vi "TCP-IP-RaspberryPi.vi"() -> ()   [LabVIEW 2021]
panel:
  out "min value":dbl
  out "max value":dbl
  in  "clear":bool
  in  "save":bool
  out "all values":dbl[](array[numeric])
  out "average":dbl format="%#_5g"
  in  "warning":dbl
  in  "danger":dbl
  out "NORMAL":bool
  out "DANGER":bool
  out "WARNING":bool
  out "Temperature":dbl(graph)
  in  "stop":bool
  out "temperature":dbl
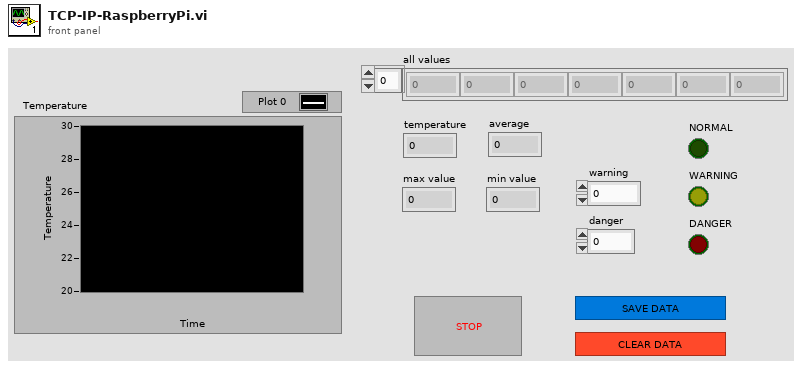
[diagram p1: front panel]
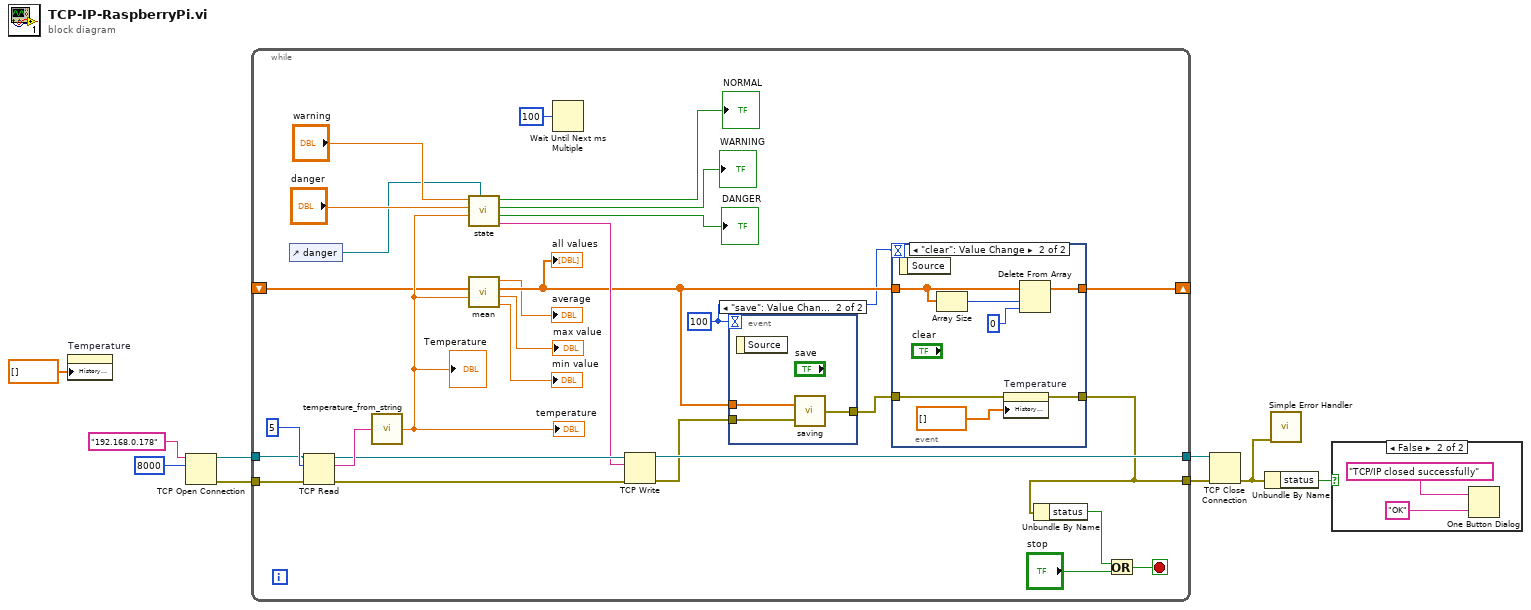
[diagram p0: block diagram]
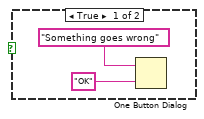
[diagram p2: hidden frame]
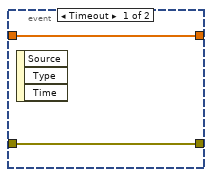
[diagram p3: hidden frame]
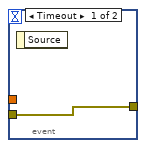
[diagram p4: hidden frame]
diagram:
  n1 = property on="Temperature" class="WFChart (strict)"("History Data"=dbl[] []) -> ()  [unwired: 2 in, 2 out]
  n2 = TCP Open Connection(address="192.168.0.178", remote port or service name=u16 8000) -> (connection ID=w6:refnum<k5>, error out=w7:errorcluster)  [unwired: 3 in]
  n3 = while {
    tunnel: w7 -> [w35]
    tunnel: w6 -> [w36]
    tunnel: [w16] -> w5
    tunnel: [w28] -> w4
    shift-right: [w18] -> _
    shift-left: _ -> [w23]
    stop <- w31 stop-if-true
    w17 = 100
    n4 = control-ref of="danger"() -> (w22:refnum<vi>)
    n5 = TCP Read(connection ID=w36, bytes to read=5, error in (no error)=w35) -> (connection ID out=w30:refnum<k5>, data out=w37:string, error out=w29:errorcluster)  [unwired: 2 in]
    n6 = call "temperature_from_string.vi"("data in"=w37) -> ("temperatura"=w24:dbl)
    "temperature" <- w24
    "Temperature" <- w24
    n7 = call "state.vi"("reference"=w22, "temperatura"=w24, "danger"="danger", "warning"="warning") -> ("string"=w26:string, "DANGER"=→"DANGER":bool, "WARNING"=→"WARNING":bool, "NORMAL"=→"NORMAL":bool)  [unwired: 1 in]
    n8 = call "mean.vi"("temperatura"=w24, "Array in"=w23) -> ("min value"=→"min value":dbl, "max value"=→"max value":dbl, "Array out"=w19:dbl[], "average"=→"average":dbl)  [unwired: 2 in]
    "all values" <- w19
    n9 = Wait Until Next ms Multiple(millisecond multiple=u32 100) -> ()  [unwired: 1 out]
    n10 = TCP Write(connection ID=w30, data in=w26, error in (no error)=w29) -> (connection ID out=w28:refnum<k5>, error out=w21:errorcluster)  [unwired: 1 in, 1 out]
    n11 = event shown="[1] \"save\": Value Change" {
      selector: _ -> [_ _]
      dyn-events: _ -> [_ _]
      timeout: w17 -> [_ _]
      tunnel: w21 -> [w48 w51]
      tunnel: [w48 w50] -> w20
      tunnel: w19 -> [_ w49]
      event Timeout {
        n12 = event-data() -> ()  [unwired: 1 in, 1 out]
      }
      event "save": Value Change {
        n13 = event-data() -> ()  [unwired: 1 in, 1 out]
        n14 = call "saving.vi"("error in (no error)"=w51, "Array in"=w49) -> ("error out"=w50:errorcluster)
      }
    }
    n15 = event shown="[1] \"clear\": Value Change" {
      selector: _ -> [_ _]
      dyn-events: _ -> [_ _]
      timeout: w17 -> [_ _]
      tunnel: w20 -> [w40 w46]
      tunnel: [w40 w41] -> w16
      tunnel: w19 -> [w39 w44]
      tunnel: [w39 w45] -> w18
      event Timeout {
        n16 = event-data() -> ()  [unwired: 1 in, 3 out]
      }
      event "clear": Value Change {
        n17 = event-data() -> ()  [unwired: 1 in, 1 out]
        n18 = Array Size(array=w44) -> (size(s)=w43:i32)
        n19 = property on="Temperature" class="WFChart (strict)"(error in=w46, "History Data"=dbl[] []) -> (error out=w41:errorcluster)  [unwired: 1 in, 1 out]
        n20 = Delete From Array(array=w44, length=w43, index=0) -> (array with subset deleted=w45:dbl[])  [unwired: 1 out]
      }
    }
    n21 = Unbundle By Name(w16) -> ("status"=w33:bool)
    n22 = Or(x=w33, y="stop") -> (x .or. y?=w31:bool)
  }
  n23 = TCP Close Connection(connection ID=w4, error in (no error)=w5) -> (error out=w2:errorcluster)  [unwired: 1 in, 1 out]
  n24 = Unbundle By Name(w2) -> ("status"=w3:bool)
  n25 = call <vilib>:"Simple Error Handler.vi"("error in (no error)"=w2) -> ()  [unwired: 4 in, 5 out]
  n26 = case shown="False" w3 {
    frame True {
      n27 = One Button Dialog(message="Something goes wrong", button name ("OK")="OK") -> ()  [unwired: 1 out]
    }
    frame False {
      n28 = One Button Dialog(message="TCP/IP closed successfully", button name ("OK")="OK") -> ()  [unwired: 1 out]
    }
  }
